vi "数组行列数.vi"(11 "数组":u32[][](array[colorbox])) -> (2 "列":i32, 3 "行":i32)   [LabVIEW 2012]
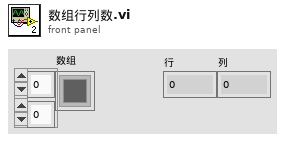
[diagram p1: front panel]
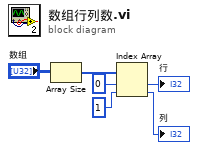
[diagram p0: block diagram]
diagram:
  n1 = Array Size(array="数组") -> (size(s)=w5:i32[])
  n2 = Index Array(array=w5, index #1=0 ("索引"), index #2=1 ("索引")) -> (element #1=→"行":i32, element #2=→"列":i32)
